vi "set_repetition_rate.vi"(8 "error in (no error)":errorcluster, 10 "repetition rate":dbl[unit], 11 "TrajectoryAK101022Resonance in":refnum<class "TrajectoryAK101022Resonance.lvclass">) -> (0 "error out":errorcluster, 3 "TrajectoryAK101022Resonance out":refnum<class "TrajectoryAK101022Resonance.lvclass">)   [LabVIEW 2010, in "TrajectoryAK101022Resonance.lvclass"]
doc: "sets the repetition rate in Hz (i.e., repetition/cycles per second)"
uses:
  TrajectoryAK101022Resonance.lvclass
  TrajectoryAK101022Resonance.lvclass/TrajectoryAK101022Resonance.ctl
  TrajectoryMG100122GenericFPGA/TrajectoryMG100122GenericFPGA/TrajectoryMG100122GenericFPGA.lvclass
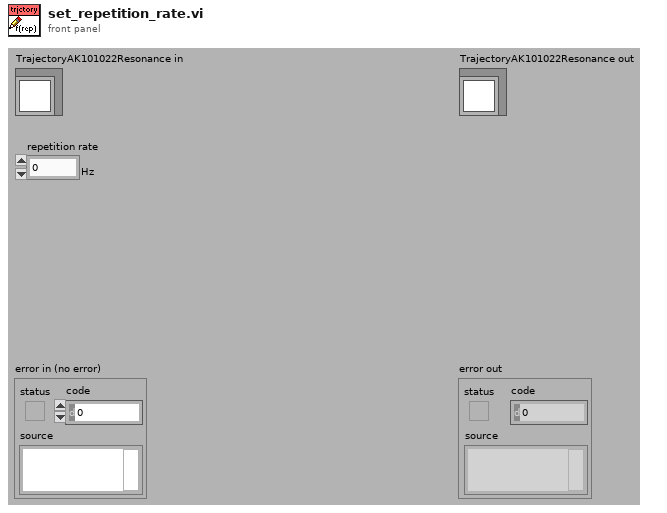
[diagram p1: front panel]
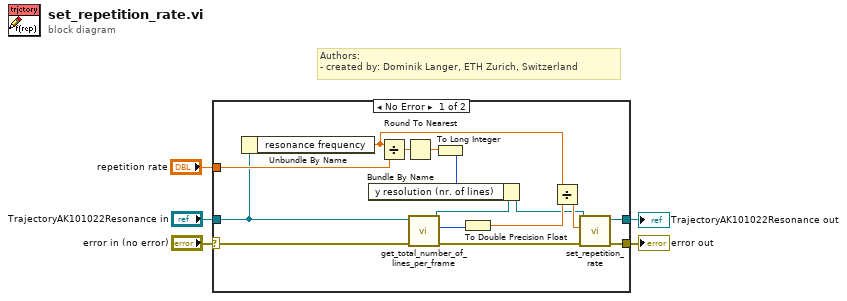
[diagram p0: block diagram]
diagram:
  # "Authors: \n- created by: Dominik Langer, ETH Zurich, Switzerland"
  n1 = case shown="No Error" "error in (no error)" {
    selector: "error in (no error)" -> [w12 w22]
    tunnel: "repetition rate" -> [w18 _]
    tunnel: "TrajectoryAK101022Resonance in" -> [w11 w21]
    tunnel: [w20 w22] -> w3
    tunnel: [w19 w21] -> w2
    frame No Error {
      n2 = Unbundle By Name(w11) -> ("resonance frequency"=w10:dbl[unit])
      n3 = Divide(x=w10, y=w18) -> (x/y=w17:dbl)
      n4 = Round To Nearest(number=w17) -> (nearest integer value=w16:dbl)
      n5 = call "get_total_number_of_lines_per_frame.vi"("error in (no error)"=w12, "TrajectoryAK101022Resonance in"=w11) -> ("error out"=w8:errorcluster, "total number of lines per frame"=w13:i32, "TrajectoryAK101022Resonance out"=w7:refnum<class "TrajectoryAK101022Resonance.lvclass">)  [unwired: 7 in]
      n6 = To Long Integer(number=w16) -> (32bit integer=w15:i32)
      n7 = Bundle By Name(cluster=w7, "y resolution (nr. of lines)"=w15) -> (w6:refnum<class "TrajectoryAK101022Resonance.lvclass">)
      n8 = To Double Precision Float(number=w13) -> (double precision float=w14:dbl)
      n9 = Divide(x=w10, y=w14) -> (x/y=w9:dbl[unit])
      n10 = call-parent "set_repetition_rate.vi"("error in (no error)"=w8, "repetition rate"=w9, "GenericTrajectory in"=w6) -> ("error out"=w20:errorcluster, "GenericTrajectory out"=w19:refnum<class "TrajectoryAK101022Resonance.lvclass">)  [unwired: 7 in]
    }
    frame Error {
    }
  }
  "error out" <- w3
  "TrajectoryAK101022Resonance out" <- w2
